vi "TurnCrank.vi"(8 "error in (no error)":errorcluster, 11 "object in":refnum<class "NoMoneyState.lvclass">) -> (0 "error out":errorcluster, 3 "object out":refnum<class "State.lvclass">)   [LabVIEW 2020, in "NoMoneyState.lvclass"]
uses:
  NoMoneyState.lvclass
  C:/Projects/OpenGDS_DesignPatterns/State1/State_class/State.lvclass
  State_class/State.lvclass
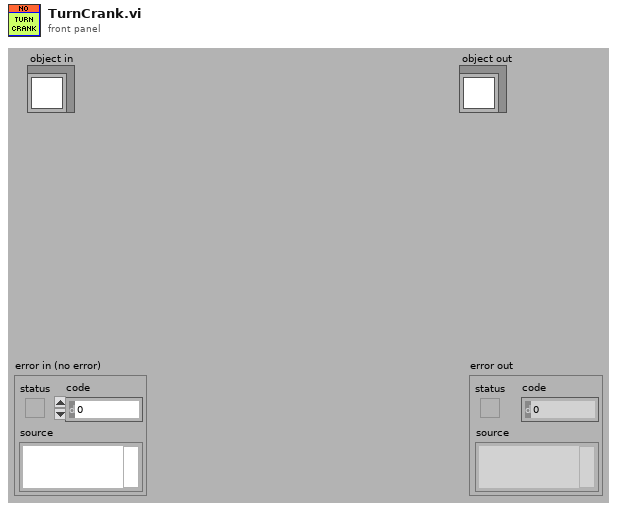
[diagram p1: front panel]
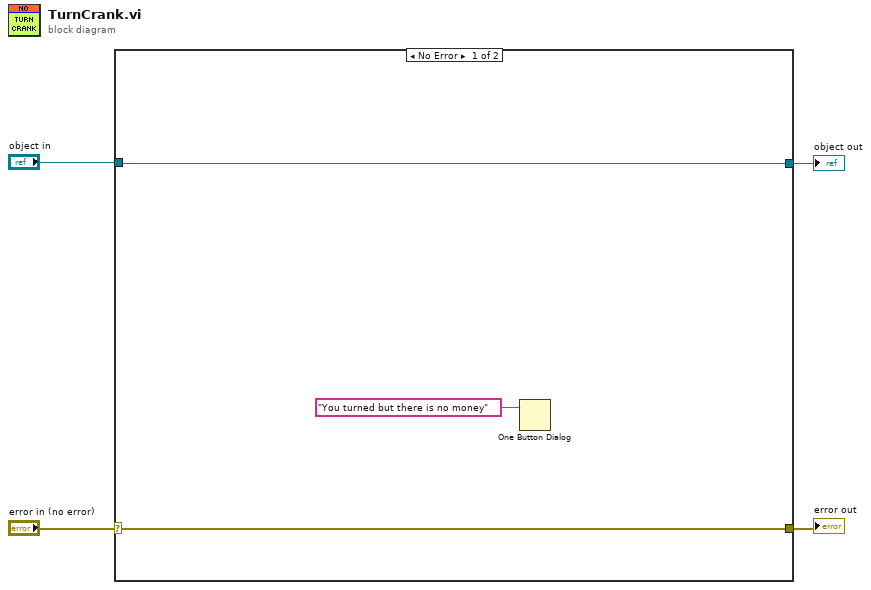
[diagram p0: block diagram]
diagram:
  n1 = case shown="No Error" "error in (no error)" {
    selector: "error in (no error)" -> [w7 w9]
    tunnel: [w7 w9] -> w3
    tunnel: [w6 w8] -> w1
    tunnel: "object in" -> [w6 w8]
    frame No Error {
      n2 = One Button Dialog(message="You turned but there is no money" ("TextIn")) -> ()  [unwired: 1 in, 1 out]
    }
    frame Error {
    }
  }
  "error out" <- w3
  "object out" <- w1
